vi "Exercises_4-8.vi"() -> ()   [LabVIEW 2014]
panel:
  out "Warning?":bool
  out "Warning Text":string
  in  "Min Temp":dbl
  in  "Max Temp":dbl
  in  "Current Temp":dbl
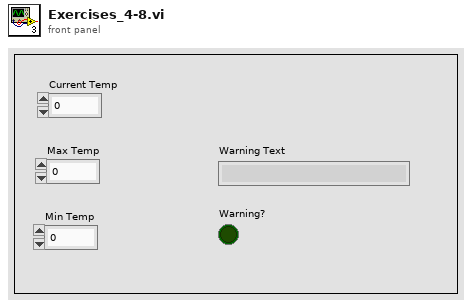
[diagram p1: front panel]
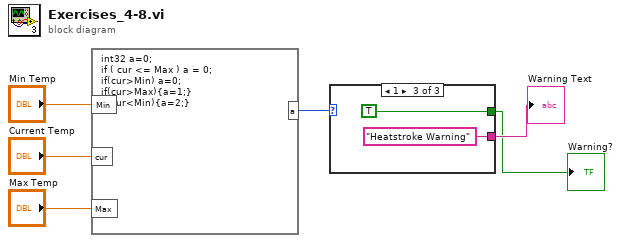
[diagram p0: block diagram]
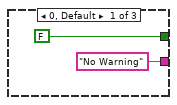
[diagram p2: hidden frame]
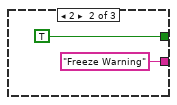
[diagram p3: hidden frame]
diagram:
  n1 = formula code="int32 a=0;\nif ( cur <= Max ) a = 0;\nif(cur>Min) a=0;\nif(cur>Max){a=1;}\nif(cur<Min){a=2;}"("Max"="Max Temp", "Min"="Min Temp", "cur"="Current Temp") -> ("a"=w3:i32)
  n2 = case shown="1" w3 {
    tunnel: ["No Warning" "Freeze Warning" "Heatstroke Warning"] -> w2
    tunnel: [FALSE TRUE TRUE] -> w1
    frame 0, Default {
    }
    frame 2 {
    }
    frame 1 {
    }
  }
  "Warning Text" <- w2
  "Warning?" <- w1
